vi "输入数据解析.vi"(0 "单个参数补充":dbl, 1 "从板号":dbl=1.0, 2 "主板二维码":string="BNET01", 3 "从板二维码":string="BNET01", 5 "主板引用":refnum<vi>, 7 "从板引用":refnum<vi>, 9 "主板选项":string="三级故障阀值", 11 "枚举":enum16{"主板", "从板"}(ring), 12 "快换":bool caption="快换写入") -> (4 "输出数组":dbl[][](array[numeric]), 6 "数组长度":dbl[](array[numeric]), 8 "循环次数":i32, 10 "命令":u32, 14 "名称":string[](array[string]), 15 "命令序号":u32[](array[numeric]))   [LabVIEW 2013] (continued)
              tunnel: [3 ("命令序号")] -> w15100
              frame 0, Default {
                n5734 = Unbundle By Name(w15110) -> ("项目信息 2"=w15111:refnum<vi>)
                n5735 = property class="Tbl (严格)"(reference=w15111) -> ("Value"=w15109:string[][])  [unwired: 1 in, 2 out]
                n5736 = Index Array(array=w15109, index (col)=1 ("禁用的索引 (列)")) -> (element=w15113:string[])  [unwired: 1 in]
                n5737 = Array Subset(array=w15113, index=2 ("索引"), length=20.0 ("y")) -> (w15114:string[])
                n5738 = Fract/Exp String To Number(string=w15114) -> (number=w15106:dbl[])  [unwired: 4 out]
                n5739 = for {
                  N: 10 -> [_]
                  tunnel: w15106 -> [w15126]
                  tunnel: [w15117] -> w15104 mode=indexing
                  i -> [w15128]
                  w15121 = 4 ("索引")
                  n5740 = Multiply(x=w15128, y=2) -> (x*y=w15125:i32)
                  n5741 = Increment(x=w15125) -> (x+1=w15124:i32)
                  n5742 = Index Array(array=w15126, index #1=w15125, index #2=w15124) -> (element #1=w15123:dbl, element #2=w15122:dbl)
                  n5743 = call "二进制解析-8.6.vi"("索引"=w15121, "数值"=w15123) -> ("低位子数组"=w15120:i32[])  [unwired: 1 in, 2 out]
                  n5744 = call "二进制解析-8.6.vi"("索引"=w15121, "数值"=w15122) -> ("低位子数组"=w15119:i32[])  [unwired: 1 in, 2 out]
                  n5745 = Insert Into Array(array=w15120, new element=w15119) -> (w15118:i32[])  [unwired: 1 in]
                  n5746 = call "数值二进制转十进制-8.6.vi"("子数组"=w15118) -> ("十进制数值"=w15117:i32)  [unwired: 4 in]
                }
              }
            }
          }
        }
        frame "温度个数" {
          n5747 = for {
            N: 1 -> [_]
            tunnel: [w15140] -> w15134 mode=indexing
            tunnel: [w15139] -> w15133 mode=indexing
            tunnel: [w15138] -> w15132 mode=indexing
            tunnel: w15131 -> [w15137]
            i -> [w15141]
            n5748 = case shown="0, 默认" w15141 {
              tunnel: w15137 -> [w15149]
              tunnel: [w15145] -> w15140
              tunnel: [4.0 ("y")] -> w15139
              tunnel: [4 ("命令序号")] -> w15138
              frame 0, Default {
                n5749 = Unbundle By Name(w15149) -> ("项目信息 2"=w15150:refnum<vi>)
                n5750 = property class="Tbl (严格)"(reference=w15150) -> ("Value"=w15148:string[][])  [unwired: 1 in, 2 out]
                n5751 = Index Array(array=w15148, index (col)=1 ("禁用的索引 (列)")) -> (element=w15152:string[])  [unwired: 1 in]
                n5752 = Array Subset(array=w15152, index=1 ("索引"), length=1.0 ("y")) -> (w15153:string[])
                n5753 = Fract/Exp String To Number(string=w15153) -> (number=w15146:dbl[])  [unwired: 4 out]
                n5754 = for {
                  N: 1 -> [_]
                  tunnel: w15146 -> [w15164] mode=indexing
                  shift-right: [w15159] -> w15145
                  shift-left: dbl[] [] -> [w15158]
                  n5755 = Quotient & Remainder(x=w15164, y=256.0) -> (x-y*floor(x/y)=w15161:dbl, floor(x/y)=w15162:dbl)
                  n5756 = Build Array(w15162, w15161, 0.0 ("元素"), 1.0 ("元素")) -> (w15160:dbl[])
                  n5757 = Insert Into Array(array=w15158, new element=w15160) -> (w15159:dbl[])  [unwired: 1 in]
                }
              }
            }
          }
        }
        frame "加热控制参数" {
          n5758 = for {
            N: 1 -> [_]
            tunnel: w15171 -> [w15175]
            tunnel: [w15178] -> w15170 mode=indexing
            tunnel: [w15177] -> w15169 mode=indexing
            tunnel: [w15176] -> w15168 mode=indexing
            tunnel: w15167 -> [w15174]
            i -> [w15179]
            n5759 = case shown="0, 默认" w15179 {
              tunnel: w15174 -> [w15199 w15205 w15246 w15290 w15334]
              tunnel: w15175 -> [_ w15209 w15250 w15294 w15339]
              tunnel: [w15185 w15210 w15255 w15299 w15338] -> w15178
              tunnel: [7.0 w15211 w15256 w15300 w15337] -> w15177
              tunnel: [u32 5 ("命令序号") u32 2 ("命令序号") u32 3 ("命令序号") u32 4 ("命令序号") u32 1 ("命令序号")] -> w15176
              frame 0, Default {
                n5760 = Unbundle By Name(w15199) -> ("加热控制参数"=w15200:refnum<vi>)
                n5761 = property class="Clust (严格)"(reference=w15200) -> ("Value"=w15198:T5)  [unwired: 1 in, 2 out]
                n5762 = Unbundle(w15198) -> ("风机开启温度"=w15193:dbl, "风机关闭温度"=w15192:dbl, "加热开启温度"=w15189:dbl, "加热关闭温度"=w15188:dbl, "风机开启温差"=w15184:dbl, "风机关闭温差"=w15183:dbl, "加热关闭温差"=w15180:dbl)
                n5763 = call "输入分辨率计算-EV05.vi"("1字节?"=TRUE, "数值 2"=w15188, "数值"=w15189, "偏移量"=-40.0, "分辨率"=1.0) -> ("高字节 2"=w15181:dbl, "高字节1"=w15182:dbl)  [unwired: 5 out]
                n5764 = call "输入分辨率计算-EV05.vi"("1字节?"=TRUE, "数值 2"=w15192, "数值"=w15193, "偏移量"=-40.0, "分辨率"=1.0) -> ("高字节 2"=w15187:dbl, "高字节1"=w15186:dbl)  [unwired: 5 out]
                n5765 = Build Array(w15186, w15187, w15184, w15183, w15182, w15181, w15180) -> (w15185:dbl[])
              }
              frame 1 {
                # "电压起始值"
                n5766 = Unbundle By Name(w15205) -> ("项目信息 2"=w15204:refnum<vi>)
                n5767 = property class="Tbl (严格)"(reference=w15204) -> ("Value"=w15203:string[][])  [unwired: 1 in, 2 out]
                n5768 = Index Array(array=w15203, index (col)=1 ("禁用的索引 (列)")) -> (element=w15217:string[])  [unwired: 1 in]
                n5769 = Multiply(x=w15209, y=6.0) -> (x*y=w15213:dbl)
                n5770 = Divide(x=w15209, y=2.0) -> (x/y=w15207:dbl)
                n5771 = Multiply(x=w15209, y=1.5) -> (x*y=w15220:dbl)
                n5772 = Array Subset(array=w15217, index=w15213, length=w15209) -> (w15215:string[])
                n5773 = Round Toward +Infinity(x=w15207) -> (ceil(x): smallest int >= x=w15206:dbl)
                n5774 = Round Toward +Infinity(x=w15220) -> (ceil(x): smallest int >= x=w15211:dbl)
                n5775 = Fract/Exp String To Number(string=w15215) -> (number=w15218:dbl[])  [unwired: 4 out]
                n5776 = for {
                  N: w15206 -> [_]
                  tunnel: w15218 -> [w15244]
                  tunnel: [w15222] -> w15221 mode=indexing
                  i -> [w15243]
                  w15234 = 256.0 ("y")
                  n5777 = Multiply(x=w15243, y=2) -> (x*y=w15241:i32)
                  n5778 = Increment(x=w15241) -> (x+1=w15240:i32)
                  n5779 = Index Array(array=w15244, index #1=w15241, index #2=w15240) -> (element #1=w15235:dbl)  [unwired: 1 out]
                  n5780 = Quotient & Remainder(x=w15235, y=w15234) -> (x-y*floor(x/y)=w15223:dbl, floor(x/y)=w15231:dbl)
                  n5781 = Quotient & Remainder(x=w15235, y=w15234) -> (x-y*floor(x/y)=w15232:dbl, floor(x/y)=w15233:dbl)
                  n5782 = call "二进制解析-8.6.vi"("索引"=4, "数值"=w15231) -> ("低位子数组"=w15227:i32[])  [unwired: 3 out]
                  n5783 = call "二进制解析-8.6.vi"("索引"=4, "数值"=w15233) -> ("低位子数组"=w15230:i32[])  [unwired: 3 out]
                  n5784 = call "二进制解析-8.6.vi"("索引"=4, "数值"=w15232) -> ("低位子数组"=w15228:i32[], "高位子数组"=w15229:i32[])  [unwired: 2 out]
                  n5785 = Insert Into Array(array=w15230, new element=w15229) -> (w15237:i32[])  [unwired: 1 in]
                  n5786 = Insert Into Array(array=w15228, new element=w15227) -> (w15226:i32[])  [unwired: 1 in]
                  n5787 = call "数值二进制转十进制-8.6.vi"("子数组"=w15226) -> ("十进制数值"=w15224:i32)  [unwired: 4 out]
                  n5788 = call "数值二进制转十进制-8.6.vi"("子数组"=w15237) -> ("十进制数值"=w15225:i32)  [unwired: 4 out]
                  n5789 = Build Array(w15225, w15224, w15223) -> (w15222:dbl[])
                }
                n5790 = Reshape Array(w15221, w15211) -> (w15210:dbl[])
              }
              frame 2 {
                # "电压起始值"
                n5791 = Unbundle By Name(w15246) -> ("项目信息 2"=w15247:refnum<vi>)
                n5792 = property class="Tbl (严格)"(reference=w15247) -> ("Value"=w15245:string[][])  [unwired: 1 in, 2 out]
                n5793 = Multiply(x=w15250, y=5.0) -> (x*y=w15248:dbl)
                n5794 = Index Array(array=w15245, index (col)=1 ("禁用的索引 (列)")) -> (element=w15261:string[])  [unwired: 1 in]
                n5795 = Multiply(x=w15250, y=7.0) -> (x*y=w15251:dbl)
                n5796 = Divide(x=w15248, y=2.0) -> (x/y=w15253:dbl)
                n5797 = Multiply(x=w15248, y=1.5) -> (x*y=w15264:dbl)
                n5798 = Array Subset(array=w15261, index=w15251, length=w15248) -> (w15259:string[])
                n5799 = Round Toward +Infinity(x=w15253) -> (ceil(x): smallest int >= x=w15252:dbl)
                n5800 = Round Toward +Infinity(x=w15264) -> (ceil(x): smallest int >= x=w15256:dbl)
                n5801 = Fract/Exp String To Number(string=w15259) -> (number=w15262:dbl[])  [unwired: 4 out]
                n5802 = for {
                  N: w15252 -> [_]
                  tunnel: w15262 -> [w15288]
                  tunnel: [w15266] -> w15265 mode=indexing
                  i -> [w15287]
                  w15278 = 256.0 ("y")
                  n5803 = Multiply(x=w15287, y=2) -> (x*y=w15285:i32)
                  n5804 = Increment(x=w15285) -> (x+1=w15284:i32)
                  n5805 = Index Array(array=w15288, index #1=w15285, index #2=w15284) -> (element #1=w15279:dbl)  [unwired: 1 out]
                  n5806 = Quotient & Remainder(x=w15279, y=w15278) -> (x-y*floor(x/y)=w15267:dbl, floor(x/y)=w15275:dbl)
                  n5807 = Quotient & Remainder(x=w15279, y=w15278) -> (x-y*floor(x/y)=w15276:dbl, floor(x/y)=w15277:dbl)
                  n5808 = call "二进制解析-8.6.vi"("索引"=4, "数值"=w15275) -> ("低位子数组"=w15271:i32[])  [unwired: 3 out]
                  n5809 = call "二进制解析-8.6.vi"("索引"=4, "数值"=w15277) -> ("低位子数组"=w15274:i32[])  [unwired: 3 out]
                  n5810 = call "二进制解析-8.6.vi"("索引"=4, "数值"=w15276) -> ("低位子数组"=w15272:i32[], "高位子数组"=w15273:i32[])  [unwired: 2 out]
                  n5811 = Insert Into Array(array=w15274, new element=w15273) -> (w15281:i32[])  [unwired: 1 in]
                  n5812 = Insert Into Array(array=w15272, new element=w15271) -> (w15270:i32[])  [unwired: 1 in]
                  n5813 = call "数值二进制转十进制-8.6.vi"("子数组"=w15270) -> ("十进制数值"=w15268:i32)  [unwired: 4 out]
                  n5814 = call "数值二进制转十进制-8.6.vi"("子数组"=w15281) -> ("十进制数值"=w15269:i32)  [unwired: 4 out]
                  n5815 = Build Array(w15269, w15268, w15267) -> (w15266:dbl[])
                }
                n5816 = Reshape Array(w15265, w15256) -> (w15255:dbl[])
              }
              frame 3 {
                # "电压起始值"
                n5817 = Unbundle By Name(w15290) -> ("项目信息 2"=w15291:refnum<vi>)
                n5818 = property class="Tbl (严格)"(reference=w15291) -> ("Value"=w15289:string[][])  [unwired: 1 in, 2 out]
                n5819 = Multiply(x=w15294, y=2.0) -> (x*y=w15292:dbl)
                n5820 = Index Array(array=w15289, index (col)=1 ("禁用的索引 (列)")) -> (element=w15305:string[])  [unwired: 1 in]
                n5821 = Multiply(x=w15294, y=11.0) -> (x*y=w15295:dbl)
                n5822 = Divide(x=w15292, y=2.0) -> (x/y=w15297:dbl)
                n5823 = Multiply(x=w15292, y=1.5) -> (x*y=w15308:dbl)
                n5824 = Array Subset(array=w15305, index=w15295, length=w15292) -> (w15303:string[])
                n5825 = Round Toward +Infinity(x=w15297) -> (ceil(x): smallest int >= x=w15296:dbl)
                n5826 = Round Toward +Infinity(x=w15308) -> (ceil(x): smallest int >= x=w15300:dbl)
                n5827 = Fract/Exp String To Number(string=w15303) -> (number=w15306:dbl[])  [unwired: 4 out]
                n5828 = for {
                  N: w15296 -> [_]
                  tunnel: w15306 -> [w15332]
                  tunnel: [w15310] -> w15309 mode=indexing
                  i -> [w15331]
                  w15322 = 256.0 ("y")
                  n5829 = Multiply(x=w15331, y=2) -> (x*y=w15329:i32)
                  n5830 = Increment(x=w15329) -> (x+1=w15328:i32)
                  n5831 = Index Array(array=w15332, index #1=w15329, index #2=w15328) -> (element #1=w15323:dbl)  [unwired: 1 out]
                  n5832 = Quotient & Remainder(x=w15323, y=w15322) -> (x-y*floor(x/y)=w15311:dbl, floor(x/y)=w15319:dbl)
                  n5833 = Quotient & Remainder(x=w15323, y=w15322) -> (x-y*floor(x/y)=w15320:dbl, floor(x/y)=w15321:dbl)
                  n5834 = call "二进制解析-8.6.vi"("索引"=4, "数值"=w15319) -> ("低位子数组"=w15315:i32[])  [unwired: 3 out]
                  n5835 = call "二进制解析-8.6.vi"("索引"=4, "数值"=w15321) -> ("低位子数组"=w15318:i32[])  [unwired: 3 out]
                  n5836 = call "二进制解析-8.6.vi"("索引"=4, "数值"=w15320) -> ("低位子数组"=w15316:i32[], "高位子数组"=w15317:i32[])  [unwired: 2 out]
                  n5837 = Insert Into Array(array=w15318, new element=w15317) -> (w15325:i32[])  [unwired: 1 in]
                  n5838 = Insert Into Array(array=w15316, new element=w15315) -> (w15314:i32[])  [unwired: 1 in]
                  n5839 = call "数值二进制转十进制-8.6.vi"("子数组"=w15314) -> ("十进制数值"=w15312:i32)  [unwired: 4 out]
                  n5840 = call "数值二进制转十进制-8.6.vi"("子数组"=w15325) -> ("十进制数值"=w15313:i32)  [unwired: 4 out]
                  n5841 = Build Array(w15313, w15312, w15311) -> (w15310:dbl[])
                }
                n5842 = Reshape Array(w15309, w15300) -> (w15299:dbl[])
              }
              frame 4 {
                n5843 = Unbundle By Name(w15334) -> ("项目信息 2"=w15335:refnum<vi>)
                n5844 = property class="Tbl (严格)"(reference=w15335) -> ("Value"=w15333:string[][])  [unwired: 1 in, 2 out]
                n5845 = Index Array(array=w15333, index (col)=1 ("禁用的索引 (列)")) -> (element=w15340:string[])  [unwired: 1 in]
                n5846 = Multiply(x=w15339, y=6.0) -> (x*y=w15337:dbl)
                n5847 = Array Subset(array=w15340, index=0 ("索引"), length=w15337) -> (w15341:string[])
                n5848 = Fract/Exp String To Number(string=w15341) -> (number=w15338:dbl[])  [unwired: 4 out]
              }
            }
          }
        }
        frame "风机开启温度" {
          n5849 = for {
            N: 1 -> [_]
            tunnel: w15351 -> [w15355]
            tunnel: [w15358] -> w15350 mode=indexing
            tunnel: [w15357] -> w15349 mode=indexing
            tunnel: [w15356] -> w15348 mode=indexing
            tunnel: w15347 -> [w15354]
            i -> [w15359]
            n5850 = case shown="0, 默认" w15359 {
              tunnel: w15354 -> [w15374 w15380 w15421 w15465 w15509]
              tunnel: w15355 -> [_ w15384 w15425 w15469 w15514]
              tunnel: [w15361 w15385 w15430 w15474 w15513] -> w15358
              tunnel: [7.0 w15386 w15431 w15475 w15512] -> w15357
              tunnel: [u32 5 ("命令序号") u32 2 ("命令序号") u32 3 ("命令序号") u32 4 ("命令序号") u32 1 ("命令序号")] -> w15356
              frame 0, Default {
                w15360 = 255 ("高字节1")
                n5851 = Unbundle By Name(w15374) -> ("加热控制参数"=w15375:refnum<vi>)
                n5852 = property class="Clust (严格)"(reference=w15375) -> ("Value"=w15373:T5)  [unwired: 1 in, 2 out]
                n5853 = Unbundle(w15373) -> ("风机开启温度"=w15368:dbl, "风机关闭温度"=w15367:dbl, "加热开启温度"=w15364:dbl, "加热关闭温度"=w15363:dbl)  [unwired: 3 out]
                n5854 = call "输入分辨率计算-EV05.vi"("1字节?"=TRUE, "数值 2"=w15363, "数值"=w15364, "偏移量"=-40.0, "分辨率"=1.0) -> ()  [unwired: 7 out]
                n5855 = call "输入分辨率计算-EV05.vi"("1字节?"=TRUE, "数值 2"=w15367, "数值"=w15368, "偏移量"=-40.0, "分辨率"=1.0) -> ("高字节1"=w15362:dbl)  [unwired: 6 out]
                n5856 = Build Array(w15362, w15360, w15360, w15360, w15360, w15360, w15360) -> (w15361:dbl[])
              }
              frame 1 {
                # "电压起始值"
                n5857 = Unbundle By Name(w15380) -> ("项目信息 2"=w15379:refnum<vi>)
                n5858 = property class="Tbl (严格)"(reference=w15379) -> ("Value"=w15378:string[][])  [unwired: 1 in, 2 out]
                n5859 = Index Array(array=w15378, index (col)=1 ("禁用的索引 (列)")) -> (element=w15392:string[])  [unwired: 1 in]
                n5860 = Multiply(x=w15384, y=6.0) -> (x*y=w15388:dbl)
                n5861 = Divide(x=w15384, y=2.0) -> (x/y=w15382:dbl)
                n5862 = Multiply(x=w15384, y=1.5) -> (x*y=w15395:dbl)
                n5863 = Array Subset(array=w15392, index=w15388, length=w15384) -> (w15390:string[])
                n5864 = Round Toward +Infinity(x=w15382) -> (ceil(x): smallest int >= x=w15381:dbl)
                n5865 = Round Toward +Infinity(x=w15395) -> (ceil(x): smallest int >= x=w15386:dbl)
                n5866 = Fract/Exp String To Number(string=w15390) -> (number=w15393:dbl[])  [unwired: 4 out]
                n5867 = for {
                  N: w15381 -> [_]
                  tunnel: w15393 -> [w15419]
                  tunnel: [w15397] -> w15396 mode=indexing
                  i -> [w15418]
                  w15409 = 256.0 ("y")
                  n5868 = Multiply(x=w15418, y=2) -> (x*y=w15416:i32)
                  n5869 = Increment(x=w15416) -> (x+1=w15415:i32)
                  n5870 = Index Array(array=w15419, index #1=w15416, index #2=w15415) -> (element #1=w15410:dbl)  [unwired: 1 out]
                  n5871 = Quotient & Remainder(x=w15410, y=w15409) -> (x-y*floor(x/y)=w15398:dbl, floor(x/y)=w15406:dbl)
                  n5872 = Quotient & Remainder(x=w15410, y=w15409) -> (x-y*floor(x/y)=w15407:dbl, floor(x/y)=w15408:dbl)
                  n5873 = call "二进制解析-8.6.vi"("索引"=4, "数值"=w15406) -> ("低位子数组"=w15402:i32[])  [unwired: 3 out]
                  n5874 = call "二进制解析-8.6.vi"("索引"=4, "数值"=w15408) -> ("低位子数组"=w15405:i32[])  [unwired: 3 out]
                  n5875 = call "二进制解析-8.6.vi"("索引"=4, "数值"=w15407) -> ("低位子数组"=w15403:i32[], "高位子数组"=w15404:i32[])  [unwired: 2 out]
                  n5876 = Insert Into Array(array=w15405, new element=w15404) -> (w15412:i32[])  [unwired: 1 in]
                  n5877 = Insert Into Array(array=w15403, new element=w15402) -> (w15401:i32[])  [unwired: 1 in]
                  n5878 = call "数值二进制转十进制-8.6.vi"("子数组"=w15401) -> ("十进制数值"=w15399:i32)  [unwired: 4 out]
                  n5879 = call "数值二进制转十进制-8.6.vi"("子数组"=w15412) -> ("十进制数值"=w15400:i32)  [unwired: 4 out]
                  n5880 = Build Array(w15400, w15399, w15398) -> (w15397:dbl[])
                }
                n5881 = Reshape Array(w15396, w15386) -> (w15385:dbl[])
              }
              frame 2 {
                # "电压起始值"
                n5882 = Unbundle By Name(w15421) -> ("项目信息 2"=w15422:refnum<vi>)
                n5883 = property class="Tbl (严格)"(reference=w15422) -> ("Value"=w15420:string[][])  [unwired: 1 in, 2 out]
                n5884 = Multiply(x=w15425, y=5.0) -> (x*y=w15423:dbl)
                n5885 = Index Array(array=w15420, index (col)=1 ("禁用的索引 (列)")) -> (element=w15436:string[])  [unwired: 1 in]
                n5886 = Multiply(x=w15425, y=7.0) -> (x*y=w15426:dbl)
                n5887 = Divide(x=w15423, y=2.0) -> (x/y=w15428:dbl)
                n5888 = Multiply(x=w15423, y=1.5) -> (x*y=w15439:dbl)
                n5889 = Array Subset(array=w15436, index=w15426, length=w15423) -> (w15434:string[])
                n5890 = Round Toward +Infinity(x=w15428) -> (ceil(x): smallest int >= x=w15427:dbl)
                n5891 = Round Toward +Infinity(x=w15439) -> (ceil(x): smallest int >= x=w15431:dbl)
                n5892 = Fract/Exp String To Number(string=w15434) -> (number=w15437:dbl[])  [unwired: 4 out]
                n5893 = for {
                  N: w15427 -> [_]
                  tunnel: w15437 -> [w15463]
                  tunnel: [w15441] -> w15440 mode=indexing
                  i -> [w15462]
                  w15453 = 256.0 ("y")
                  n5894 = Multiply(x=w15462, y=2) -> (x*y=w15460:i32)
                  n5895 = Increment(x=w15460) -> (x+1=w15459:i32)
                  n5896 = Index Array(array=w15463, index #1=w15460, index #2=w15459) -> (element #1=w15454:dbl)  [unwired: 1 out]
                  n5897 = Quotient & Remainder(x=w15454, y=w15453) -> (x-y*floor(x/y)=w15442:dbl, floor(x/y)=w15450:dbl)
                  n5898 = Quotient & Remainder(x=w15454, y=w15453) -> (x-y*floor(x/y)=w15451:dbl, floor(x/y)=w15452:dbl)
                  n5899 = call "二进制解析-8.6.vi"("索引"=4, "数值"=w15450) -> ("低位子数组"=w15446:i32[])  [unwired: 3 out]
                  n5900 = call "二进制解析-8.6.vi"("索引"=4, "数值"=w15452) -> ("低位子数组"=w15449:i32[])  [unwired: 3 out]
                  n5901 = call "二进制解析-8.6.vi"("索引"=4, "数值"=w15451) -> ("低位子数组"=w15447:i32[], "高位子数组"=w15448:i32[])  [unwired: 2 out]
                  n5902 = Insert Into Array(array=w15449, new element=w15448) -> (w15456:i32[])  [unwired: 1 in]
                  n5903 = Insert Into Array(array=w15447, new element=w15446) -> (w15445:i32[])  [unwired: 1 in]
                  n5904 = call "数值二进制转十进制-8.6.vi"("子数组"=w15445) -> ("十进制数值"=w15443:i32)  [unwired: 4 out]
                  n5905 = call "数值二进制转十进制-8.6.vi"("子数组"=w15456) -> ("十进制数值"=w15444:i32)  [unwired: 4 out]
                  n5906 = Build Array(w15444, w15443, w15442) -> (w15441:dbl[])
                }
                n5907 = Reshape Array(w15440, w15431) -> (w15430:dbl[])
              }
              frame 3 {
                # "电压起始值"
                n5908 = Unbundle By Name(w15465) -> ("项目信息 2"=w15466:refnum<vi>)
                n5909 = property class="Tbl (严格)"(reference=w15466) -> ("Value"=w15464:string[][])  [unwired: 1 in, 2 out]
                n5910 = Multiply(x=w15469, y=2.0) -> (x*y=w15467:dbl)
                n5911 = Index Array(array=w15464, index (col)=1 ("禁用的索引 (列)")) -> (element=w15480:string[])  [unwired: 1 in]
                n5912 = Multiply(x=w15469, y=11.0) -> (x*y=w15470:dbl)
                n5913 = Divide(x=w15467, y=2.0) -> (x/y=w15472:dbl)
                n5914 = Multiply(x=w15467, y=1.5) -> (x*y=w15483:dbl)
                n5915 = Array Subset(array=w15480, index=w15470, length=w15467) -> (w15478:string[])
                n5916 = Round Toward +Infinity(x=w15472) -> (ceil(x): smallest int >= x=w15471:dbl)
                n5917 = Round Toward +Infinity(x=w15483) -> (ceil(x): smallest int >= x=w15475:dbl)
                n5918 = Fract/Exp String To Number(string=w15478) -> (number=w15481:dbl[])  [unwired: 4 out]
                n5919 = for {
                  N: w15471 -> [_]
                  tunnel: w15481 -> [w15507]
                  tunnel: [w15485] -> w15484 mode=indexing
                  i -> [w15506]
                  w15497 = 256.0 ("y")
                  n5920 = Multiply(x=w15506, y=2) -> (x*y=w15504:i32)
                  n5921 = Increment(x=w15504) -> (x+1=w15503:i32)
                  n5922 = Index Array(array=w15507, index #1=w15504, index #2=w15503) -> (element #1=w15498:dbl)  [unwired: 1 out]
                  n5923 = Quotient & Remainder(x=w15498, y=w15497) -> (x-y*floor(x/y)=w15486:dbl, floor(x/y)=w15494:dbl)
                  n5924 = Quotient & Remainder(x=w15498, y=w15497) -> (x-y*floor(x/y)=w15495:dbl, floor(x/y)=w15496:dbl)
                  n5925 = call "二进制解析-8.6.vi"("索引"=4, "数值"=w15494) -> ("低位子数组"=w15490:i32[])  [unwired: 3 out]
                  n5926 = call "二进制解析-8.6.vi"("索引"=4, "数值"=w15496) -> ("低位子数组"=w15493:i32[])  [unwired: 3 out]
                  n5927 = call "二进制解析-8.6.vi"("索引"=4, "数值"=w15495) -> ("低位子数组"=w15491:i32[], "高位子数组"=w15492:i32[])  [unwired: 2 out]
                  n5928 = Insert Into Array(array=w15493, new element=w15492) -> (w15500:i32[])  [unwired: 1 in]
                  n5929 = Insert Into Array(array=w15491, new element=w15490) -> (w15489:i32[])  [unwired: 1 in]
                  n5930 = call "数值二进制转十进制-8.6.vi"("子数组"=w15489) -> ("十进制数值"=w15487:i32)  [unwired: 4 out]
                  n5931 = call "数值二进制转十进制-8.6.vi"("子数组"=w15500) -> ("十进制数值"=w15488:i32)  [unwired: 4 out]
                  n5932 = Build Array(w15488, w15487, w15486) -> (w15485:dbl[])
                }
                n5933 = Reshape Array(w15484, w15475) -> (w15474:dbl[])
              }
              frame 4 {
                n5934 = Unbundle By Name(w15509) -> ("项目信息 2"=w15510:refnum<vi>)
                n5935 = property class="Tbl (严格)"(reference=w15510) -> ("Value"=w15508:string[][])  [unwired: 1 in, 2 out]
                n5936 = Index Array(array=w15508, index (col)=1 ("禁用的索引 (列)")) -> (element=w15515:string[])  [unwired: 1 in]
                n5937 = Multiply(x=w15514, y=6.0) -> (x*y=w15512:dbl)
                n5938 = Array Subset(array=w15515, index=0 ("索引"), length=w15512) -> (w15516:string[])
                n5939 = Fract/Exp String To Number(string=w15516) -> (number=w15513:dbl[])  [unwired: 4 out]
              }
            }
          }
        }
        frame "风机关闭温度" {
          n5940 = for {
            N: 1 -> [_]
            tunnel: w15526 -> [w15530]
            tunnel: [w15533] -> w15525 mode=indexing
            tunnel: [w15532] -> w15524 mode=indexing
            tunnel: [w15531] -> w15523 mode=indexing
            tunnel: w15522 -> [w15529]
            i -> [w15534]
            n5941 = case shown="0, 默认" w15534 {
              tunnel: w15529 -> [w15549 w15555 w15596 w15640 w15684]
              tunnel: w15530 -> [_ w15559 w15600 w15644 w15689]
              tunnel: [w15537 w15560 w15605 w15649 w15688] -> w15533
              tunnel: [7.0 w15561 w15606 w15650 w15687] -> w15532
              tunnel: [u32 5 ("命令序号") u32 2 ("命令序号") u32 3 ("命令序号") u32 4 ("命令序号") u32 1 ("命令序号")] -> w15531
              frame 0, Default {
                w15535 = 255 ("高字节1")
                n5942 = Unbundle By Name(w15549) -> ("加热控制参数"=w15550:refnum<vi>)
                n5943 = property class="Clust (严格)"(reference=w15550) -> ("Value"=w15548:T5)  [unwired: 1 in, 2 out]
                n5944 = Unbundle(w15548) -> ("风机开启温度"=w15543:dbl, "风机关闭温度"=w15542:dbl, "加热开启温度"=w15539:dbl, "加热关闭温度"=w15538:dbl)  [unwired: 3 out]
                n5945 = call "输入分辨率计算-EV05.vi"("1字节?"=TRUE, "数值 2"=w15538, "数值"=w15539, "偏移量"=-40.0, "分辨率"=1.0) -> ()  [unwired: 7 out]
                n5946 = call "输入分辨率计算-EV05.vi"("1字节?"=TRUE, "数值 2"=w15542, "数值"=w15543, "偏移量"=-40.0, "分辨率"=1.0) -> ("高字节 2"=w15536:dbl)  [unwired: 6 out]
                n5947 = Build Array(w15535, w15536, w15535, w15535, w15535, w15535, w15535) -> (w15537:dbl[])
              }
              frame 1 {
                # "电压起始值"
                n5948 = Unbundle By Name(w15555) -> ("项目信息 2"=w15554:refnum<vi>)
                n5949 = property class="Tbl (严格)"(reference=w15554) -> ("Value"=w15553:string[][])  [unwired: 1 in, 2 out]
                n5950 = Index Array(array=w15553, index (col)=1 ("禁用的索引 (列)")) -> (element=w15567:string[])  [unwired: 1 in]
                n5951 = Multiply(x=w15559, y=6.0) -> (x*y=w15563:dbl)
                n5952 = Divide(x=w15559, y=2.0) -> (x/y=w15557:dbl)
                n5953 = Multiply(x=w15559, y=1.5) -> (x*y=w15570:dbl)
                n5954 = Array Subset(array=w15567, index=w15563, length=w15559) -> (w15565:string[])
                n5955 = Round Toward +Infinity(x=w15557) -> (ceil(x): smallest int >= x=w15556:dbl)
                n5956 = Round Toward +Infinity(x=w15570) -> (ceil(x): smallest int >= x=w15561:dbl)
                n5957 = Fract/Exp String To Number(string=w15565) -> (number=w15568:dbl[])  [unwired: 4 out]
                n5958 = for {
                  N: w15556 -> [_]
                  tunnel: w15568 -> [w15594]
                  tunnel: [w15572] -> w15571 mode=indexing
                  i -> [w15593]
                  w15584 = 256.0 ("y")
                  n5959 = Multiply(x=w15593, y=2) -> (x*y=w15591:i32)
                  n5960 = Increment(x=w15591) -> (x+1=w15590:i32)
                  n5961 = Index Array(array=w15594, index #1=w15591, index #2=w15590) -> (element #1=w15585:dbl)  [unwired: 1 out]
                  n5962 = Quotient & Remainder(x=w15585, y=w15584) -> (x-y*floor(x/y)=w15573:dbl, floor(x/y)=w15581:dbl)
                  n5963 = Quotient & Remainder(x=w15585, y=w15584) -> (x-y*floor(x/y)=w15582:dbl, floor(x/y)=w15583:dbl)
                  n5964 = call "二进制解析-8.6.vi"("索引"=4, "数值"=w15581) -> ("低位子数组"=w15577:i32[])  [unwired: 3 out]
                  n5965 = call "二进制解析-8.6.vi"("索引"=4, "数值"=w15583) -> ("低位子数组"=w15580:i32[])  [unwired: 3 out]
                  n5966 = call "二进制解析-8.6.vi"("索引"=4, "数值"=w15582) -> ("低位子数组"=w15578:i32[], "高位子数组"=w15579:i32[])  [unwired: 2 out]
                  n5967 = Insert Into Array(array=w15580, new element=w15579) -> (w15587:i32[])  [unwired: 1 in]
                  n5968 = Insert Into Array(array=w15578, new element=w15577) -> (w15576:i32[])  [unwired: 1 in]
                  n5969 = call "数值二进制转十进制-8.6.vi"("子数组"=w15576) -> ("十进制数值"=w15574:i32)  [unwired: 4 out]
                  n5970 = call "数值二进制转十进制-8.6.vi"("子数组"=w15587) -> ("十进制数值"=w15575:i32)  [unwired: 4 out]
                  n5971 = Build Array(w15575, w15574, w15573) -> (w15572:dbl[])
                }
                n5972 = Reshape Array(w15571, w15561) -> (w15560:dbl[])
              }
              frame 2 {
                # "电压起始值"
                n5973 = Unbundle By Name(w15596) -> ("项目信息 2"=w15597:refnum<vi>)
                n5974 = property class="Tbl (严格)"(reference=w15597) -> ("Value"=w15595:string[][])  [unwired: 1 in, 2 out]
                n5975 = Multiply(x=w15600, y=5.0) -> (x*y=w15598:dbl)
                n5976 = Index Array(array=w15595, index (col)=1 ("禁用的索引 (列)")) -> (element=w15611:string[])  [unwired: 1 in]
                n5977 = Multiply(x=w15600, y=7.0) -> (x*y=w15601:dbl)
                n5978 = Divide(x=w15598, y=2.0) -> (x/y=w15603:dbl)
                n5979 = Multiply(x=w15598, y=1.5) -> (x*y=w15614:dbl)
                n5980 = Array Subset(array=w15611, index=w15601, length=w15598) -> (w15609:string[])
                n5981 = Round Toward +Infinity(x=w15603) -> (ceil(x): smallest int >= x=w15602:dbl)
                n5982 = Round Toward +Infinity(x=w15614) -> (ceil(x): smallest int >= x=w15606:dbl)
                n5983 = Fract/Exp String To Number(string=w15609) -> (number=w15612:dbl[])  [unwired: 4 out]
                n5984 = for {
                  N: w15602 -> [_]
                  tunnel: w15612 -> [w15638]
                  tunnel: [w15616] -> w15615 mode=indexing
                  i -> [w15637]
                  w15628 = 256.0 ("y")
                  n5985 = Multiply(x=w15637, y=2) -> (x*y=w15635:i32)
                  n5986 = Increment(x=w15635) -> (x+1=w15634:i32)
                  n5987 = Index Array(array=w15638, index #1=w15635, index #2=w15634) -> (element #1=w15629:dbl)  [unwired: 1 out]
                  n5988 = Quotient & Remainder(x=w15629, y=w15628) -> (x-y*floor(x/y)=w15617:dbl, floor(x/y)=w15625:dbl)
                  n5989 = Quotient & Remainder(x=w15629, y=w15628) -> (x-y*floor(x/y)=w15626:dbl, floor(x/y)=w15627:dbl)
                  n5990 = call "二进制解析-8.6.vi"("索引"=4, "数值"=w15625) -> ("低位子数组"=w15621:i32[])  [unwired: 3 out]
                  n5991 = call "二进制解析-8.6.vi"("索引"=4, "数值"=w15627) -> ("低位子数组"=w15624:i32[])  [unwired: 3 out]
                  n5992 = call "二进制解析-8.6.vi"("索引"=4, "数值"=w15626) -> ("低位子数组"=w15622:i32[], "高位子数组"=w15623:i32[])  [unwired: 2 out]
                  n5993 = Insert Into Array(array=w15624, new element=w15623) -> (w15631:i32[])  [unwired: 1 in]
                  n5994 = Insert Into Array(array=w15622, new element=w15621) -> (w15620:i32[])  [unwired: 1 in]
                  n5995 = call "数值二进制转十进制-8.6.vi"("子数组"=w15620) -> ("十进制数值"=w15618:i32)  [unwired: 4 out]
                  n5996 = call "数值二进制转十进制-8.6.vi"("子数组"=w15631) -> ("十进制数值"=w15619:i32)  [unwired: 4 out]
                  n5997 = Build Array(w15619, w15618, w15617) -> (w15616:dbl[])
                }
                n5998 = Reshape Array(w15615, w15606) -> (w15605:dbl[])
              }
              frame 3 {
                # "电压起始值"
                n5999 = Unbundle By Name(w15640) -> ("项目信息 2"=w15641:refnum<vi>)
                n6000 = property class="Tbl (严格)"(reference=w15641) -> ("Value"=w15639:string[][])  [unwired: 1 in, 2 out]
                n6001 = Multiply(x=w15644, y=2.0) -> (x*y=w15642:dbl)
                n6002 = Index Array(array=w15639, index (col)=1 ("禁用的索引 (列)")) -> (element=w15655:string[])  [unwired: 1 in]
                n6003 = Multiply(x=w15644, y=11.0) -> (x*y=w15645:dbl)
                n6004 = Divide(x=w15642, y=2.0) -> (x/y=w15647:dbl)
                n6005 = Multiply(x=w15642, y=1.5) -> (x*y=w15658:dbl)
                n6006 = Array Subset(array=w15655, index=w15645, length=w15642) -> (w15653:string[])
                n6007 = Round Toward +Infinity(x=w15647) -> (ceil(x): smallest int >= x=w15646:dbl)
                n6008 = Round Toward +Infinity(x=w15658) -> (ceil(x): smallest int >= x=w15650:dbl)
                n6009 = Fract/Exp String To Number(string=w15653) -> (number=w15656:dbl[])  [unwired: 4 out]
                n6010 = for {
                  N: w15646 -> [_]
                  tunnel: w15656 -> [w15682]
                  tunnel: [w15660] -> w15659 mode=indexing
                  i -> [w15681]
                  w15672 = 256.0 ("y")
                  n6011 = Multiply(x=w15681, y=2) -> (x*y=w15679:i32)
                  n6012 = Increment(x=w15679) -> (x+1=w15678:i32)
                  n6013 = Index Array(array=w15682, index #1=w15679, index #2=w15678) -> (element #1=w15673:dbl)  [unwired: 1 out]
                  n6014 = Quotient & Remainder(x=w15673, y=w15672) -> (x-y*floor(x/y)=w15661:dbl, floor(x/y)=w15669:dbl)
                  n6015 = Quotient & Remainder(x=w15673, y=w15672) -> (x-y*floor(x/y)=w15670:dbl, floor(x/y)=w15671:dbl)
                  n6016 = call "二进制解析-8.6.vi"("索引"=4, "数值"=w15669) -> ("低位子数组"=w15665:i32[])  [unwired: 3 out]
                  n6017 = call "二进制解析-8.6.vi"("索引"=4, "数值"=w15671) -> ("低位子数组"=w15668:i32[])  [unwired: 3 out]
                  n6018 = call "二进制解析-8.6.vi"("索引"=4, "数值"=w15670) -> ("低位子数组"=w15666:i32[], "高位子数组"=w15667:i32[])  [unwired: 2 out]
                  n6019 = Insert Into Array(array=w15668, new element=w15667) -> (w15675:i32[])  [unwired: 1 in]
                  n6020 = Insert Into Array(array=w15666, new element=w15665) -> (w15664:i32[])  [unwired: 1 in]
                  n6021 = call "数值二进制转十进制-8.6.vi"("子数组"=w15664) -> ("十进制数值"=w15662:i32)  [unwired: 4 out]
                  n6022 = call "数值二进制转十进制-8.6.vi"("子数组"=w15675) -> ("十进制数值"=w15663:i32)  [unwired: 4 out]
                  n6023 = Build Array(w15663, w15662, w15661) -> (w15660:dbl[])
                }
                n6024 = Reshape Array(w15659, w15650) -> (w15649:dbl[])
              }
              frame 4 {
                n6025 = Unbundle By Name(w15684) -> ("项目信息 2"=w15685:refnum<vi>)
                n6026 = property class="Tbl (严格)"(reference=w15685) -> ("Value"=w15683:string[][])  [unwired: 1 in, 2 out]
                n6027 = Index Array(array=w15683, index (col)=1 ("禁用的索引 (列)")) -> (element=w15690:string[])  [unwired: 1 in]
                n6028 = Multiply(x=w15689, y=6.0) -> (x*y=w15687:dbl)
                n6029 = Array Subset(array=w15690, index=0 ("索引"), length=w15687) -> (w15691:string[])
                n6030 = Fract/Exp String To Number(string=w15691) -> (number=w15688:dbl[])  [unwired: 4 out]
              }
            }
          }
        }
        frame "加热开启温度" {
          n6031 = for {
            N: 1 -> [_]
            tunnel: w15701 -> [w15705]
            tunnel: [w15708] -> w15700 mode=indexing
            tunnel: [w15707] -> w15699 mode=indexing
            tunnel: [w15706] -> w15698 mode=indexing
            tunnel: w15697 -> [w15704]
            i -> [w15709]
            n6032 = case shown="0, 默认" w15709 {
              tunnel: w15704 -> [w15724 w15730 w15771 w15815 w15859]
              tunnel: w15705 -> [_ w15734 w15775 w15819 w15864]
              tunnel: [w15712 w15735 w15780 w15824 w15863] -> w15708
              tunnel: [7.0 w15736 w15781 w15825 w15862] -> w15707
              tunnel: [u32 5 ("命令序号") u32 2 ("命令序号") u32 3 ("命令序号") u32 4 ("命令序号") u32 1 ("命令序号")] -> w15706
              frame 0, Default {
                w15710 = 255 ("高字节1")
                n6033 = Unbundle By Name(w15724) -> ("加热控制参数"=w15725:refnum<vi>)
                n6034 = property class="Clust (严格)"(reference=w15725) -> ("Value"=w15723:T5)  [unwired: 1 in, 2 out]
                n6035 = Unbundle(w15723) -> ("风机开启温度"=w15718:dbl, "风机关闭温度"=w15717:dbl, "加热开启温度"=w15714:dbl, "加热关闭温度"=w15713:dbl)  [unwired: 3 out]
                n6036 = call "输入分辨率计算-EV05.vi"("1字节?"=TRUE, "数值 2"=w15713, "数值"=w15714, "偏移量"=-40.0, "分辨率"=1.0) -> ("高字节1"=w15711:dbl)  [unwired: 6 out]
                n6037 = call "输入分辨率计算-EV05.vi"("1字节?"=TRUE, "数值 2"=w15717, "数值"=w15718, "偏移量"=-40.0, "分辨率"=1.0) -> ()  [unwired: 7 out]
                n6038 = Build Array(w15710, w15710, w15710, w15710, w15711, w15710, w15710) -> (w15712:dbl[])
              }
              frame 1 {
                # "电压起始值"
                n6039 = Unbundle By Name(w15730) -> ("项目信息 2"=w15729:refnum<vi>)
                n6040 = property class="Tbl (严格)"(reference=w15729) -> ("Value"=w15728:string[][])  [unwired: 1 in, 2 out]
                n6041 = Index Array(array=w15728, index (col)=1 ("禁用的索引 (列)")) -> (element=w15742:string[])  [unwired: 1 in]
                n6042 = Multiply(x=w15734, y=6.0) -> (x*y=w15738:dbl)
                n6043 = Divide(x=w15734, y=2.0) -> (x/y=w15732:dbl)
                n6044 = Multiply(x=w15734, y=1.5) -> (x*y=w15745:dbl)
                n6045 = Array Subset(array=w15742, index=w15738, length=w15734) -> (w15740:string[])
                n6046 = Round Toward +Infinity(x=w15732) -> (ceil(x): smallest int >= x=w15731:dbl)
                n6047 = Round Toward +Infinity(x=w15745) -> (ceil(x): smallest int >= x=w15736:dbl)
                n6048 = Fract/Exp String To Number(string=w15740) -> (number=w15743:dbl[])  [unwired: 4 out]
                n6049 = for {
                  N: w15731 -> [_]
                  tunnel: w15743 -> [w15769]
                  tunnel: [w15747] -> w15746 mode=indexing
                  i -> [w15768]
                  w15759 = 256.0 ("y")
                  n6050 = Multiply(x=w15768, y=2) -> (x*y=w15766:i32)
                  n6051 = Increment(x=w15766) -> (x+1=w15765:i32)
                  n6052 = Index Array(array=w15769, index #1=w15766, index #2=w15765) -> (element #1=w15760:dbl)  [unwired: 1 out]
                  n6053 = Quotient & Remainder(x=w15760, y=w15759) -> (x-y*floor(x/y)=w15748:dbl, floor(x/y)=w15756:dbl)
                  n6054 = Quotient & Remainder(x=w15760, y=w15759) -> (x-y*floor(x/y)=w15757:dbl, floor(x/y)=w15758:dbl)
                  n6055 = call "二进制解析-8.6.vi"("索引"=4, "数值"=w15756) -> ("低位子数组"=w15752:i32[])  [unwired: 3 out]
                  n6056 = call "二进制解析-8.6.vi"("索引"=4, "数值"=w15758) -> ("低位子数组"=w15755:i32[])  [unwired: 3 out]
                  n6057 = call "二进制解析-8.6.vi"("索引"=4, "数值"=w15757) -> ("低位子数组"=w15753:i32[], "高位子数组"=w15754:i32[])  [unwired: 2 out]
                  n6058 = Insert Into Array(array=w15755, new element=w15754) -> (w15762:i32[])  [unwired: 1 in]
                  n6059 = Insert Into Array(array=w15753, new element=w15752) -> (w15751:i32[])  [unwired: 1 in]
                  n6060 = call "数值二进制转十进制-8.6.vi"("子数组"=w15751) -> ("十进制数值"=w15749:i32)  [unwired: 4 out]
                  n6061 = call "数值二进制转十进制-8.6.vi"("子数组"=w15762) -> ("十进制数值"=w15750:i32)  [unwired: 4 out]
                  n6062 = Build Array(w15750, w15749, w15748) -> (w15747:dbl[])
                }
                n6063 = Reshape Array(w15746, w15736) -> (w15735:dbl[])
              }
              frame 2 {
                # "电压起始值"
                n6064 = Unbundle By Name(w15771) -> ("项目信息 2"=w15772:refnum<vi>)
                n6065 = property class="Tbl (严格)"(reference=w15772) -> ("Value"=w15770:string[][])  [unwired: 1 in, 2 out]
                n6066 = Multiply(x=w15775, y=5.0) -> (x*y=w15773:dbl)
                n6067 = Index Array(array=w15770, index (col)=1 ("禁用的索引 (列)")) -> (element=w15786:string[])  [unwired: 1 in]
                n6068 = Multiply(x=w15775, y=7.0) -> (x*y=w15776:dbl)
                n6069 = Divide(x=w15773, y=2.0) -> (x/y=w15778:dbl)
                n6070 = Multiply(x=w15773, y=1.5) -> (x*y=w15789:dbl)
                n6071 = Array Subset(array=w15786, index=w15776, length=w15773) -> (w15784:string[])
                n6072 = Round Toward +Infinity(x=w15778) -> (ceil(x): smallest int >= x=w15777:dbl)
                n6073 = Round Toward +Infinity(x=w15789) -> (ceil(x): smallest int >= x=w15781:dbl)
                n6074 = Fract/Exp String To Number(string=w15784) -> (number=w15787:dbl[])  [unwired: 4 out]
                n6075 = for {
                  N: w15777 -> [_]
                  tunnel: w15787 -> [w15813]
                  tunnel: [w15791] -> w15790 mode=indexing
                  i -> [w15812]
                  w15803 = 256.0 ("y")
                  n6076 = Multiply(x=w15812, y=2) -> (x*y=w15810:i32)
                  n6077 = Increment(x=w15810) -> (x+1=w15809:i32)
                  n6078 = Index Array(array=w15813, index #1=w15810, index #2=w15809) -> (element #1=w15804:dbl)  [unwired: 1 out]
                  n6079 = Quotient & Remainder(x=w15804, y=w15803) -> (x-y*floor(x/y)=w15792:dbl, floor(x/y)=w15800:dbl)
                  n6080 = Quotient & Remainder(x=w15804, y=w15803) -> (x-y*floor(x/y)=w15801:dbl, floor(x/y)=w15802:dbl)
                  n6081 = call "二进制解析-8.6.vi"("索引"=4, "数值"=w15800) -> ("低位子数组"=w15796:i32[])  [unwired: 3 out]
                  n6082 = call "二进制解析-8.6.vi"("索引"=4, "数值"=w15802) -> ("低位子数组"=w15799:i32[])  [unwired: 3 out]
                  n6083 = call "二进制解析-8.6.vi"("索引"=4, "数值"=w15801) -> ("低位子数组"=w15797:i32[], "高位子数组"=w15798:i32[])  [unwired: 2 out]
                  n6084 = Insert Into Array(array=w15799, new element=w15798) -> (w15806:i32[])  [unwired: 1 in]
                  n6085 = Insert Into Array(array=w15797, new element=w15796) -> (w15795:i32[])  [unwired: 1 in]
                  n6086 = call "数值二进制转十进制-8.6.vi"("子数组"=w15795) -> ("十进制数值"=w15793:i32)  [unwired: 4 out]
                  n6087 = call "数值二进制转十进制-8.6.vi"("子数组"=w15806) -> ("十进制数值"=w15794:i32)  [unwired: 4 out]
                  n6088 = Build Array(w15794, w15793, w15792) -> (w15791:dbl[])
                }
                n6089 = Reshape Array(w15790, w15781) -> (w15780:dbl[])
              }
              frame 3 {
                # "电压起始值"
                n6090 = Unbundle By Name(w15815) -> ("项目信息 2"=w15816:refnum<vi>)
                n6091 = property class="Tbl (严格)"(reference=w15816) -> ("Value"=w15814:string[][])  [unwired: 1 in, 2 out]
                n6092 = Multiply(x=w15819, y=2.0) -> (x*y=w15817:dbl)
                n6093 = Index Array(array=w15814, index (col)=1 ("禁用的索引 (列)")) -> (element=w15830:string[])  [unwired: 1 in]
                n6094 = Multiply(x=w15819, y=11.0) -> (x*y=w15820:dbl)
                n6095 = Divide(x=w15817, y=2.0) -> (x/y=w15822:dbl)
                n6096 = Multiply(x=w15817, y=1.5) -> (x*y=w15833:dbl)
                n6097 = Array Subset(array=w15830, index=w15820, length=w15817) -> (w15828:string[])
                n6098 = Round Toward +Infinity(x=w15822) -> (ceil(x): smallest int >= x=w15821:dbl)
                n6099 = Round Toward +Infinity(x=w15833) -> (ceil(x): smallest int >= x=w15825:dbl)
                n6100 = Fract/Exp String To Number(string=w15828) -> (number=w15831:dbl[])  [unwired: 4 out]
                n6101 = for {
                  N: w15821 -> [_]
                  tunnel: w15831 -> [w15857]
                  tunnel: [w15835] -> w15834 mode=indexing
                  i -> [w15856]
                  w15847 = 256.0 ("y")
                  n6102 = Multiply(x=w15856, y=2) -> (x*y=w15854:i32)
                  n6103 = Increment(x=w15854) -> (x+1=w15853:i32)
                  n6104 = Index Array(array=w15857, index #1=w15854, index #2=w15853) -> (element #1=w15848:dbl)  [unwired: 1 out]
                  n6105 = Quotient & Remainder(x=w15848, y=w15847) -> (x-y*floor(x/y)=w15836:dbl, floor(x/y)=w15844:dbl)
                  n6106 = Quotient & Remainder(x=w15848, y=w15847) -> (x-y*floor(x/y)=w15845:dbl, floor(x/y)=w15846:dbl)
                  n6107 = call "二进制解析-8.6.vi"("索引"=4, "数值"=w15844) -> ("低位子数组"=w15840:i32[])  [unwired: 3 out]
                  n6108 = call "二进制解析-8.6.vi"("索引"=4, "数值"=w15846) -> ("低位子数组"=w15843:i32[])  [unwired: 3 out]
                  n6109 = call "二进制解析-8.6.vi"("索引"=4, "数值"=w15845) -> ("低位子数组"=w15841:i32[], "高位子数组"=w15842:i32[])  [unwired: 2 out]
                  n6110 = Insert Into Array(array=w15843, new element=w15842) -> (w15850:i32[])  [unwired: 1 in]
                  n6111 = Insert Into Array(array=w15841, new element=w15840) -> (w15839:i32[])  [unwired: 1 in]
                  n6112 = call "数值二进制转十进制-8.6.vi"("子数组"=w15839) -> ("十进制数值"=w15837:i32)  [unwired: 4 out]
                  n6113 = call "数值二进制转十进制-8.6.vi"("子数组"=w15850) -> ("十进制数值"=w15838:i32)  [unwired: 4 out]
                  n6114 = Build Array(w15838, w15837, w15836) -> (w15835:dbl[])
                }
                n6115 = Reshape Array(w15834, w15825) -> (w15824:dbl[])
              }
              frame 4 {
                n6116 = Unbundle By Name(w15859) -> ("项目信息 2"=w15860:refnum<vi>)
                n6117 = property class="Tbl (严格)"(reference=w15860) -> ("Value"=w15858:string[][])  [unwired: 1 in, 2 out]
                n6118 = Index Array(array=w15858, index (col)=1 ("禁用的索引 (列)")) -> (element=w15865:string[])  [unwired: 1 in]
                n6119 = Multiply(x=w15864, y=6.0) -> (x*y=w15862:dbl)
                n6120 = Array Subset(array=w15865, index=0 ("索引"), length=w15862) -> (w15866:string[])
                n6121 = Fract/Exp String To Number(string=w15866) -> (number=w15863:dbl[])  [unwired: 4 out]
              }
            }
          }
        }
        frame "加热关闭温度" {
          n6122 = for {
            N: 1 -> [_]
            tunnel: w15876 -> [w15880]
            tunnel: [w15883] -> w15875 mode=indexing
            tunnel: [w15882] -> w15874 mode=indexing
            tunnel: [w15881] -> w15873 mode=indexing
            tunnel: w15872 -> [w15879]
            i -> [w15884]
            n6123 = case shown="0, 默认" w15884 {
              tunnel: w15879 -> [w15899 w15905 w15946 w15990 w16034]
              tunnel: w15880 -> [_ w15909 w15950 w15994 w16039]
              tunnel: [w15887 w15910 w15955 w15999 w16038] -> w15883
              tunnel: [7.0 w15911 w15956 w16000 w16037] -> w15882
              tunnel: [u32 5 ("命令序号") u32 2 ("命令序号") u32 3 ("命令序号") u32 4 ("命令序号") u32 1 ("命令序号")] -> w15881
              frame 0, Default {
                w15885 = 255 ("高字节1")
                n6124 = Unbundle By Name(w15899) -> ("加热控制参数"=w15900:refnum<vi>)
                n6125 = property class="Clust (严格)"(reference=w15900) -> ("Value"=w15898:T5)  [unwired: 1 in, 2 out]
                n6126 = Unbundle(w15898) -> ("风机开启温度"=w15893:dbl, "风机关闭温度"=w15892:dbl, "加热开启温度"=w15889:dbl, "加热关闭温度"=w15888:dbl)  [unwired: 3 out]
                n6127 = call "输入分辨率计算-EV05.vi"("1字节?"=TRUE, "数值 2"=w15888, "数值"=w15889, "偏移量"=-40.0, "分辨率"=1.0) -> ("高字节 2"=w15886:dbl)  [unwired: 6 out]
                n6128 = call "输入分辨率计算-EV05.vi"("1字节?"=TRUE, "数值 2"=w15892, "数值"=w15893, "偏移量"=-40.0, "分辨率"=1.0) -> ()  [unwired: 7 out]
                n6129 = Build Array(w15885, w15885, w15885, w15885, w15885, w15886, w15885) -> (w15887:dbl[])
              }
              frame 1 {
                # "电压起始值"
                n6130 = Unbundle By Name(w15905) -> ("项目信息 2"=w15904:refnum<vi>)
                n6131 = property class="Tbl (严格)"(reference=w15904) -> ("Value"=w15903:string[][])  [unwired: 1 in, 2 out]
                n6132 = Index Array(array=w15903, index (col)=1 ("禁用的索引 (列)")) -> (element=w15917:string[])  [unwired: 1 in]
                n6133 = Multiply(x=w15909, y=6.0) -> (x*y=w15913:dbl)
                n6134 = Divide(x=w15909, y=2.0) -> (x/y=w15907:dbl)
                n6135 = Multiply(x=w15909, y=1.5) -> (x*y=w15920:dbl)
                n6136 = Array Subset(array=w15917, index=w15913, length=w15909) -> (w15915:string[])
                n6137 = Round Toward +Infinity(x=w15907) -> (ceil(x): smallest int >= x=w15906:dbl)
                n6138 = Round Toward +Infinity(x=w15920) -> (ceil(x): smallest int >= x=w15911:dbl)
                n6139 = Fract/Exp String To Number(string=w15915) -> (number=w15918:dbl[])  [unwired: 4 out]
                n6140 = for {
                  N: w15906 -> [_]
                  tunnel: w15918 -> [w15944]
                  tunnel: [w15922] -> w15921 mode=indexing
                  i -> [w15943]
                  w15934 = 256.0 ("y")
                  n6141 = Multiply(x=w15943, y=2) -> (x*y=w15941:i32)
                  n6142 = Increment(x=w15941) -> (x+1=w15940:i32)
                  n6143 = Index Array(array=w15944, index #1=w15941, index #2=w15940) -> (element #1=w15935:dbl)  [unwired: 1 out]
                  n6144 = Quotient & Remainder(x=w15935, y=w15934) -> (x-y*floor(x/y)=w15923:dbl, floor(x/y)=w15931:dbl)
                  n6145 = Quotient & Remainder(x=w15935, y=w15934) -> (x-y*floor(x/y)=w15932:dbl, floor(x/y)=w15933:dbl)
                  n6146 = call "二进制解析-8.6.vi"("索引"=4, "数值"=w15931) -> ("低位子数组"=w15927:i32[])  [unwired: 3 out]
                  n6147 = call "二进制解析-8.6.vi"("索引"=4, "数值"=w15933) -> ("低位子数组"=w15930:i32[])  [unwired: 3 out]
                  n6148 = call "二进制解析-8.6.vi"("索引"=4, "数值"=w15932) -> ("低位子数组"=w15928:i32[], "高位子数组"=w15929:i32[])  [unwired: 2 out]
                  n6149 = Insert Into Array(array=w15930, new element=w15929) -> (w15937:i32[])  [unwired: 1 in]
                  n6150 = Insert Into Array(array=w15928, new element=w15927) -> (w15926:i32[])  [unwired: 1 in]
                  n6151 = call "数值二进制转十进制-8.6.vi"("子数组"=w15926) -> ("十进制数值"=w15924:i32)  [unwired: 4 out]
                  n6152 = call "数值二进制转十进制-8.6.vi"("子数组"=w15937) -> ("十进制数值"=w15925:i32)  [unwired: 4 out]
                  n6153 = Build Array(w15925, w15924, w15923) -> (w15922:dbl[])
                }
                n6154 = Reshape Array(w15921, w15911) -> (w15910:dbl[])
              }
              frame 2 {
                # "电压起始值"
                n6155 = Unbundle By Name(w15946) -> ("项目信息 2"=w15947:refnum<vi>)
                n6156 = property class="Tbl (严格)"(reference=w15947) -> ("Value"=w15945:string[][])  [unwired: 1 in, 2 out]
                n6157 = Multiply(x=w15950, y=5.0) -> (x*y=w15948:dbl)
                n6158 = Index Array(array=w15945, index (col)=1 ("禁用的索引 (列)")) -> (element=w15961:string[])  [unwired: 1 in]
                n6159 = Multiply(x=w15950, y=7.0) -> (x*y=w15951:dbl)
                n6160 = Divide(x=w15948, y=2.0) -> (x/y=w15953:dbl)
                n6161 = Multiply(x=w15948, y=1.5) -> (x*y=w15964:dbl)
                n6162 = Array Subset(array=w15961, index=w15951, length=w15948) -> (w15959:string[])
                n6163 = Round Toward +Infinity(x=w15953) -> (ceil(x): smallest int >= x=w15952:dbl)
                n6164 = Round Toward +Infinity(x=w15964) -> (ceil(x): smallest int >= x=w15956:dbl)
                n6165 = Fract/Exp String To Number(string=w15959) -> (number=w15962:dbl[])  [unwired: 4 out]
                n6166 = for {
                  N: w15952 -> [_]
                  tunnel: w15962 -> [w15988]
                  tunnel: [w15966] -> w15965 mode=indexing
                  i -> [w15987]
                  w15978 = 256.0 ("y")
                  n6167 = Multiply(x=w15987, y=2) -> (x*y=w15985:i32)
                  n6168 = Increment(x=w15985) -> (x+1=w15984:i32)
                  n6169 = Index Array(array=w15988, index #1=w15985, index #2=w15984) -> (element #1=w15979:dbl)  [unwired: 1 out]
                  n6170 = Quotient & Remainder(x=w15979, y=w15978) -> (x-y*floor(x/y)=w15967:dbl, floor(x/y)=w15975:dbl)
                  n6171 = Quotient & Remainder(x=w15979, y=w15978) -> (x-y*floor(x/y)=w15976:dbl, floor(x/y)=w15977:dbl)
                  n6172 = call "二进制解析-8.6.vi"("索引"=4, "数值"=w15975) -> ("低位子数组"=w15971:i32[])  [unwired: 3 out]
                  n6173 = call "二进制解析-8.6.vi"("索引"=4, "数值"=w15977) -> ("低位子数组"=w15974:i32[])  [unwired: 3 out]
                  n6174 = call "二进制解析-8.6.vi"("索引"=4, "数值"=w15976) -> ("低位子数组"=w15972:i32[], "高位子数组"=w15973:i32[])  [unwired: 2 out]
                  n6175 = Insert Into Array(array=w15974, new element=w15973) -> (w15981:i32[])  [unwired: 1 in]
                  n6176 = Insert Into Array(array=w15972, new element=w15971) -> (w15970:i32[])  [unwired: 1 in]
                  n6177 = call "数值二进制转十进制-8.6.vi"("子数组"=w15970) -> ("十进制数值"=w15968:i32)  [unwired: 4 out]
                  n6178 = call "数值二进制转十进制-8.6.vi"("子数组"=w15981) -> ("十进制数值"=w15969:i32)  [unwired: 4 out]
                  n6179 = Build Array(w15969, w15968, w15967) -> (w15966:dbl[])
                }
                n6180 = Reshape Array(w15965, w15956) -> (w15955:dbl[])
              }
              frame 3 {
                # "电压起始值"
